vi "Generate Bins.vi"(1 "min":dbl format="%0.2f", 2 "max":dbl format="%0.2f", 3 "inclusion":enum32{"lower", "upper"}(ring), 4 "# bins":i32, 5 "Bins":T2(array[cluster]) {"upper" format="%0.2f"; "lower" format="%0.2f"}, 6 "Input Data":dbl[](array[numeric]) format="%0.2f") -> (0 "Bins out":T1(array[cluster]) {"upper" format="%0.2f"; "lower" format="%0.2f"})   [LabVIEW 2020, in "NI_PtbyPt.lvlib"]
uses:
  NI_PtbyPt.lvlib
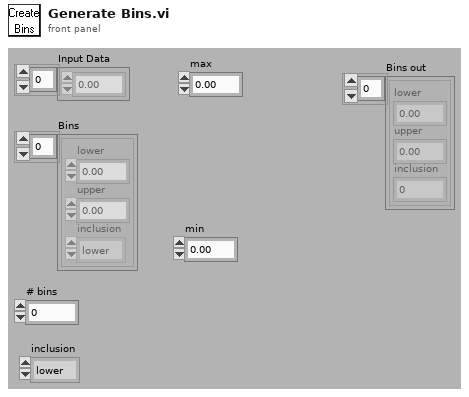
[diagram p1: front panel]
types:
  T1 = cluster{"lower":dbl, "upper":dbl, "inclusion":u32}[]
  T2 = cluster{"lower":dbl, "upper":dbl, "inclusion":enum32{"lower", "upper", "both", "neither"}}[]
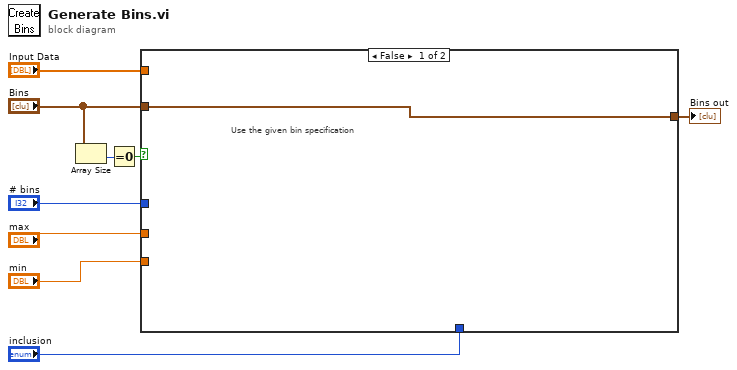
[diagram p0: block diagram]
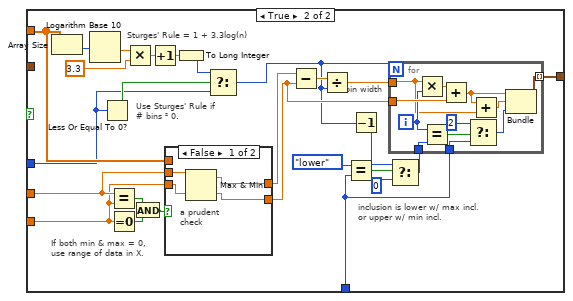
[diagram p2: hidden frame]
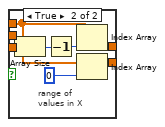
[diagram p3: hidden frame]
diagram:
  n1 = Array Size(array="Bins") -> (size(s)=w1:i32)
  n2 = Equal To 0?(x=w1) -> (x = 0?=w2:bool)
  n3 = case shown="False" w2 {
    tunnel: [w10 w16] -> w3
    tunnel: "Input Data" -> [_ w33]
    tunnel: "Bins" -> [w10 _]
    tunnel: "inclusion" -> [_ w14]
    tunnel: "max" -> [_ w13]
    tunnel: "min" -> [_ w12]
    tunnel: "# bins" -> [_ w11]
    frame False {
      # "Use the given bin specification"
    }
    frame True {
      # "inclusion is lower w/ max incl.\nor upper w/ min incl."
      # "bin width"
      # "Use Sturges' Rule if\n# bins ² 0."
      # "If both min & max = 0,\nuse range of data in X."
      # "Sturges' Rule = 1 + 3.3log(n)"
      n4 = Array Size(array=w33) -> (size(s)=w31:i32)
      n5 = Logarithm Base 10(1:w31) -> (0:w29:dbl)
      n6 = Less Or Equal To 0?(x=w11) -> (x <= 0?=w32:bool)
      n7 = Equal?(x=w13, y=w12) -> (x = y?=w35:bool)
      n8 = Equal To 0?(x=w12) -> (x = 0?=w36:bool)
      n9 = Multiply(x=w29, y=3.3) -> (x*y=w28:dbl)
      n10 = And(x=w35, y=w36) -> (x .and. y?=w34:bool)
      n11 = Increment(x=w28) -> (x+1=w27:dbl)
      n12 = case shown="False" w34 {
        tunnel: w33 -> [_ w58]
        tunnel: [w52 w56] -> w19
        tunnel: [w50 w54] -> w18
        tunnel: w13 -> [w51 _]
        tunnel: w12 -> [w49 _]
        frame False {
          # "a prudent\ncheck"
          n13 = Max & Min(x=w51, y=w49) -> (max(x,y)=w52:dbl, min(x,y)=w50:dbl)
        }
        frame True {
          # "range of \nvalues in X"
          n14 = Array Size(array=w58) -> (size(s)=w57:i32)
          n15 = Decrement(x=w57) -> (x-1=w53:i32)
          n16 = Index Array(array=w58, index=w53) -> (element=w56:dbl)
          n17 = Index Array(array=w58, index=0 ("Index")) -> (element=w54:dbl)
        }
      }
      n18 = To Long Integer(number=w27) -> (32bit integer=w26:i32)
      n19 = Select(t=w26, s=w32, f=w11) -> (s? t:f=w17:i32)
      n20 = Subtract(x=w19, y=w18) -> (x-y=w25:dbl)
      n21 = Divide(x=w25, y=w17) -> (x/y=w20:dbl)
      n22 = Equal?(x=enum32{"lower", "upper"}."lower" ("inclusion"), y=w14) -> (x = y?=w24:bool)
      n23 = Decrement(x=w17) -> (x-1=w23:i32)
      n24 = Select(t=w23, s=w24, f=0) -> (s? t:f=w21:i32)
      n25 = for {
        N: w17 -> [_]
        tunnel: w20 -> [w37]
        tunnel: w14 -> [w41]
        tunnel: [w48] -> w16 mode=indexing
        tunnel: w18 -> [w45]
        tunnel: w21 -> [w38]
        i -> [w43]
        n26 = Multiply(x=w37, y=w43) -> (x*y=w46:dbl)
        n27 = Equal?(x=w43, y=w38) -> (x = y?=w42:bool)
        n28 = Add(x=w46, y=w45) -> (x+y=w44:dbl)
        n29 = Select(t=2, s=w42, f=w41) -> (s? t:f=w40:u32)
        n30 = Add(x=w44, y=w37) -> (x+y=w47:dbl)
        n31 = Bundle(w44, w47, "inclusion"=w40) -> (w48:cluster{dbl, dbl, "inclusion":u32})  [unwired: 1 in]
      }
    }
  }
  "Bins out" <- w3
